vi "Reanimate.vi"(8 "Error In":errorcluster) -> (0 "Error Out":errorcluster)   [LabVIEW 2018, in "Tests.lvlib" / "Toolkit.lvlib"]
uses:
  Toolkit.lvlib
  src/Toolkit/Toolkit.lvlib
  <vilib>/addons/_JKI Toolkits/Caraya/classes/Test/Test.lvclass
  <vilib>/addons/_JKI Toolkits/Caraya/classes/Assert/Assert.lvclass
  Tests.lvlib
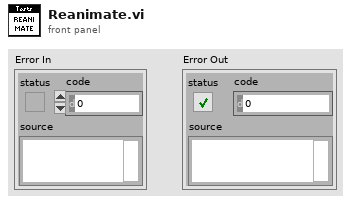
[diagram p1: front panel]
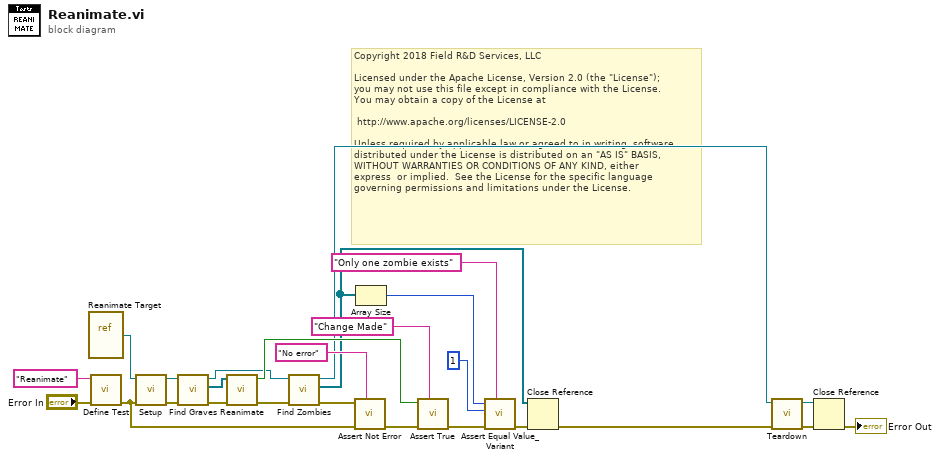
[diagram p0: block diagram]
diagram:
  # "Copyright 2018 Field R&D Services, LLC\n\nLicensed under the Apache License, Version 2.0 (the \"License\");\nyou may not use this file except in compliance with the License.\nYou may obtain a copy of the License at\n\n\thttp://www.apache.org/licenses/LICENSE-2.0\n\nUnless required by applicable law or agreed to in writing, software\ndistributed under the License is distributed on an \"AS IS\" BASIS,\nWITHOUT WARRANTIES OR CONDITIONS OF ANY KIND, either \nexpress  or implied.  See the License for the specific language \ngoverning permissions and limitations under the License."
  n1 = vi-ref "Reanimate Target.vi"() -> (w15:refnum<vi>)
  n2 = call <vilib>:"Define Test.vi"("error in (no error)"="Error In", "Label (VI Title)"="Reanimate") -> ("error out"=w6:errorcluster)  [unwired: 9 in]
  n3 = call "Setup.vi"("Error In"=w6, "VI In"=w15) -> ("Error Out"=w5:errorcluster, "VI Out"=w7:refnum<vi>)  [unwired: 8 in]
  n4 = call "Find Graves.vi"("Error In"=w5, "VI In"=w7) -> ("Error Out"=w11:errorcluster, "Graves"=w9:refnum<vi>[], "VI Out"=w10:refnum<vi>)  [unwired: 7 in]
  n5 = call "Reanimate.vi"("Error In"=w11, "Graves"=w9) -> ("Error Out"=w26:errorcluster, "Change Made?"=w13:bool)  [unwired: 8 in]
  n6 = call "Find Zombies.vi"("Error In"=w26, "VI In"=w10) -> ("Error Out"=w21:errorcluster, "Graves"=w8:refnum<vi>[], "VI Out"=w2:refnum<vi>)  [unwired: 7 in]
  n7 = call <vilib>:"Assert Not Error.vi"("Label"="No error", "error in (no error)"=w6, "Not Error?"=w21) -> ("error out"=w23:errorcluster)  [unwired: 8 in]
  n8 = Array Size(array=w8) -> (size(s)=w20:i32)
  n9 = call <vilib>:"Assert True.vi"("Label"="Change Made", "error in (no error)"=w23, "True?"=w13) -> ("error out"=w14:errorcluster)  [unwired: 8 in]
  n10 = call <vilib>:"Assert Equal Value_Variant.vi"("Label"="Only one zombie exists", "error in (no error)"=w14, "Y"=1 ("size(s)"), "X"=w20) -> ("error out"=w17:errorcluster)  [unwired: 7 in]
  n11 = Close Reference(reference=w8, error in (no error)=w17) -> (error out=w4:errorcluster)
  n12 = call "Teardown.vi"("Error In"=w4, "VI In"=w2) -> ("Error Out"=w3:errorcluster, "VI Out"=w1:refnum<vi>)  [unwired: 8 in]
  n13 = Close Reference(reference=w1, error in (no error)=w3) -> (error out=→"Error Out":errorcluster)
